vi "get Disappearing.vi"(11 "Element in":refnum<class "Element.lvclass">) -> (3 "Disappearing":bool)   [LabVIEW 2021, in "Element.lvclass"]
uses:
  Element.lvclass
  Element.lvclass/Element.ctl
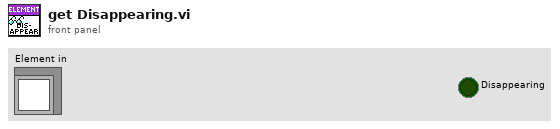
[diagram p1: front panel]
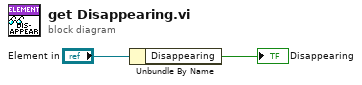
[diagram p0: block diagram]
diagram:
  n1 = Unbundle By Name("Element in") -> ("Disappearing"=→"Disappearing":bool)
